vi "_Raise WebMessageReceived.vi"(4 "Display State In":T1, 5 "Event Data":cluster{"sender":refnum<k24>, "e":refnum<k24>}, 6 "Control Ref":refnum<k24>, 7 "Event Common Data":T2) -> ()   [LabVIEW 2020, in "WebView2 Control.xctl"]
uses:
  WebView2 Control.xctl
  E:/Labview/LV 2020/Libs/WebView2/LV-WebView2/Source/Libs/Microsoft.Web.WebView2.Core.dll
  Libs/Microsoft.Web.WebView2.Core.dll
  Events.ctl
  Navigation Event Data.ctl
  Source Changed Event Data.ctl
  Navigation Start Event Data.ctl
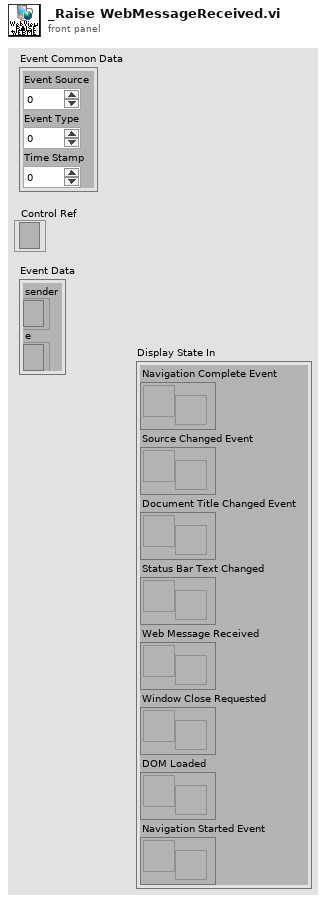
[diagram p1: front panel]
types:
  T1 = typedef "WebView2 Control.xctl/Events.ctl" = cluster{"Navigation Complete Event":refnum<user-event>, "Source Changed Event":refnum<user-event>, "Document Title Changed Event":refnum<user-event>, "Status Bar Text Changed":refnum<user-event>, "Web Message Received":refnum<user-event>, "Window Close Requested":refnum<user-event>, "DOM Loaded":refnum<user-event>, "Navigation Started Event":refnum<user-event>}
  T2 = cluster{"Event Source":i32, "Event Type":u32, "Time Stamp":u32}
  T3 = cluster{"Source":string, "WebMessageAsJson":string}
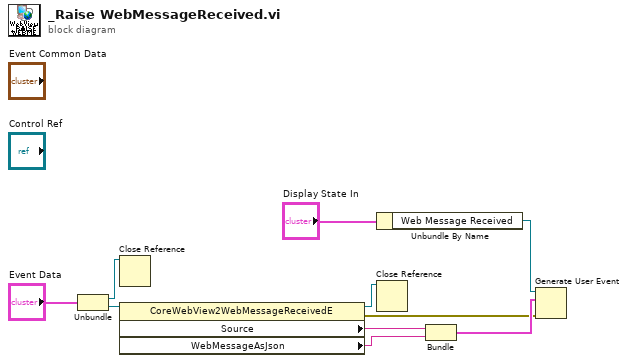
[diagram p0: block diagram]
diagram:
  n1 = Unbundle("Event Data") -> ("sender"=w2:refnum<k24>, "e"=w7:refnum<k24>)
  n2 = Close Reference(reference=w2) -> ()  [unwired: 1 in, 1 out]
  n3 = property class="CoreWebView2WebMessageReceivedE"(reference=w7) -> (reference out=w1:refnum<k24>, error out=w3:errorcluster, "Source"=w6:string, "WebMessageAsJson"=w5:string)  [unwired: 1 in]
  n4 = Unbundle By Name("Display State In") -> ("Web Message Received"=w8:refnum<user-event>)
  n5 = Close Reference(reference=w1) -> ()  [unwired: 1 in, 1 out]
  n6 = Bundle("Source"=w6, "WebMessageAsJson"=w5) -> (w4:T3)  [unwired: 1 in]
  n7 = Generate User Event(user event=w8, event data cluster=w4, error in=w3) -> ()  [unwired: 1 in, 2 out]
